vi "ReadColumnRgbaU64.vi"(8 "error in":errorcluster, 10 "Column":i32, 11 "Image Reference In":T2) -> (0 "error out":errorcluster, 2 "Pixel Column":T1[](array[typedef]), 3 "Image Reference Out":T2)   [LabVIEW 2020, in "OpenLvVision_Image.lvlib" / "DataAccess.lvlib"]
doc: "Returns the values of an pixel column."
uses:
  DataAccess.lvlib
  Management/TypeDef/Image.ctl
  <vilib>/Utility/error.llb/Error Cluster From Error Code.vi
  <vilib>/ErrorRing/Error Ring.xnode
  Management/Management.lvlib
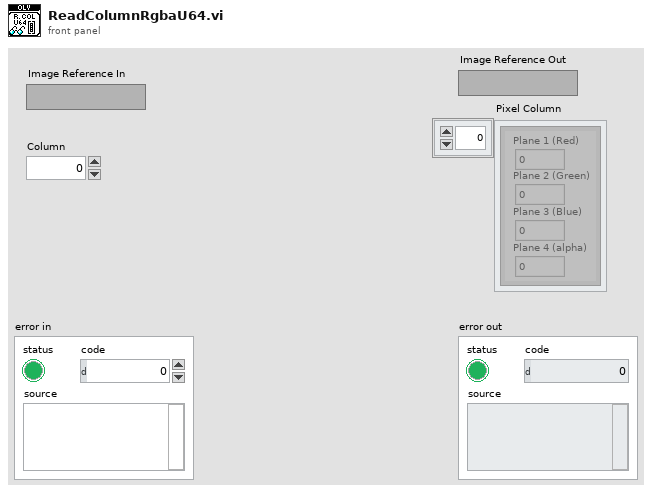
[diagram p1: front panel]
types:
  T1 = typedef "Color (U64)" = cluster{"Plane 3 (Blue)":u16, "Plane 2 (Green)":u16, "Plane 1 (Red)":u16, "Plane 4 (alpha)":u16}
  T2 = typedef "OpenLvVision_Image.lvlib/Management.lvlib/Image.ctl" = refnum<image>
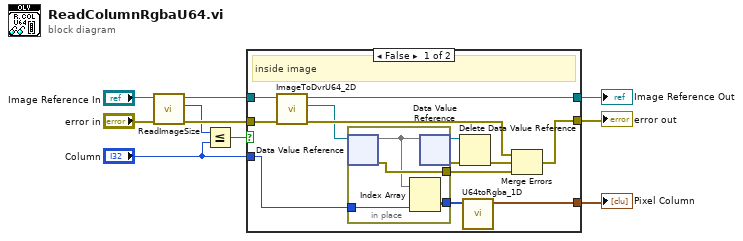
[diagram p0: block diagram]
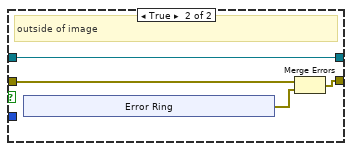
[diagram p2: hidden frame]
diagram:
  n1 = call "ReadImageSize.vi"("error in"="error in", "Image Reference In"="Image Reference In") -> ("error out"=w9:errorcluster, "Width"=w1:i32, "Image Reference Out"=w10:T2)  [unwired: 6 in, 1 out]
  n2 = Less Or Equal?(x=w1, y="Column") -> (x <= y?=w4:bool)
  n3 = case shown="False" w4 {
    tunnel: w10 -> [w23 w29]
    tunnel: w9 -> [w22 w31]
    tunnel: [w21 w29] -> w6
    tunnel: [w14 w28] -> w5
    tunnel: [w11 _] -> w2
    tunnel: "Column" -> [w13 _]
    frame False {
      # "inside image"
      n4 = call "ImageToDvrU64_2D.vi"("error in"=w22, "Image Reference In"=w23) -> ("error out"=w16:errorcluster, "EDVR 2D U64"=w15:refnum<data-value>, "Image Reference Out"=w21:T2)  [unwired: 6 in, 1 out]
      n5 = in-place {
        in-place-border: [w27] -> w19
        in-place-border: [w25] -> w12
        in-place-border: w13 -> [w24]
        n6 = in-place-dvr #1(w15) -> (w26:u64[][], w27:errorcluster)
        n7 = Index Array(array=w26, index (col)=w24) -> (element=w25:u64[])  [unwired: 1 in]
        n8 = in-place-dvr #1(w26) -> (w17:refnum<data-value>, w18:errorcluster)
      }
      n9 = Delete Data Value Reference(data value reference=w17, error in=w18) -> (error out=w20:errorcluster)  [unwired: 1 out]
      n10 = call "U64toRgba_1D.vi"("U64"=w12) -> ("Rgba"=w11:T1[])  [unwired: 10 in]
      n11 = Merge Errors(w16, w20, w19) -> (w14:errorcluster)
    }
    frame True {
      # "outside of image"
      n12 = xnode "Error Ring"() -> ("error out"=w30:errorcluster)
      n13 = Merge Errors(w31, w30) -> (w28:errorcluster)
    }
  }
  "error out" <- w5
  "Image Reference Out" <- w6
  "Pixel Column" <- w2
